vi "Parse GGA Sentence.vi"(7 "date override":timestamp format="%<%x>T", 8 "error in (no error)":errorcluster, 11 "GGA sentence":string) -> (0 "error out":errorcluster, 3 "GGA data":T1 {"DGPS station ID number"."station ID number" min=0.0; "fix quality"."quality" items=["Invalid", "GPS Fix", "DGPS Fix", "PPS Fix", "Real Time Kinematic", "Float RTK", "Estimated", "Manual Input Mode", "Simulation Mode"]; "time of fix"."time (UTC)" format="%^<%.3X\n%x>T"})   [LabVIEW 2017, in "NMEA API.lvlib"]
doc: "Returns data contained in a particular type of NMEA sentence. The input sentence you specify must include valid NMEA formatting and end with a carriage return and line feed, or \\r\\n. You must manually select the polymorphic instance to use."
uses:
  <vilib>/robotics/Protocols/NMEA/NMEA API.lvlib
  <vilib>/robotics/Protocols/NMEA/typedefs/GGA Data.ctl
  <vilib>/robotics/Utilities/NI_Robotics Utilities.lvlib
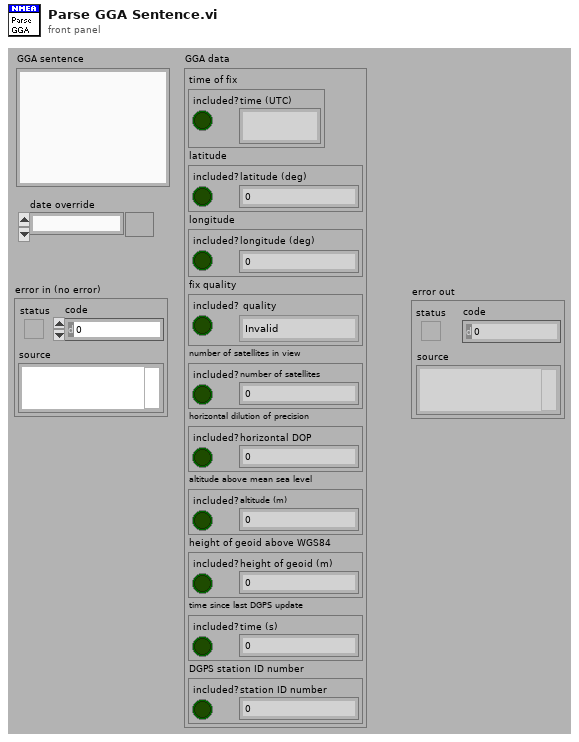
[diagram p1: front panel]
types:
  T1 = typedef "NMEA API.lvlib/GGA Data.ctl" = cluster{"time of fix":cluster{"included?":bool, "time (UTC)":timestamp}, "latitude":cluster{"included?":bool, "latitude (deg)":dbl}, "longitude":cluster{"included?":bool, "longitude (deg)":dbl}, "fix quality":cluster{"included?":bool, "quality":u16}, "number of satellites in view":cluster{"included?":bool, "number of satellites":i8}, "horizontal dilution of precision":cluster{"included?":bool, "horizontal DOP":dbl}, "altitude above mean sea level":cluster{"included?":bool, "altitude (m)":dbl}, "height of geoid above WGS84":cluster{"included?":bool, "height of geoid (m)":dbl}, "time since last DGPS update":cluster{"included?":bool, "time (s)":dbl}, "DGPS station ID number":cluster{"included?":bool, "station ID number":dbl}}
  T2 = cluster{"Valid?":bool, "Number of Satellites":i8}
  T3 = typedef "LVDateTimeRec.ctl" = cluster{"fractional second":dbl, "second":i32, "minute":i32, "hour":i32, "day of month":i32, "month":i32, "year":i32, "day of week":i32, "day of year":i32, "DST":i32}
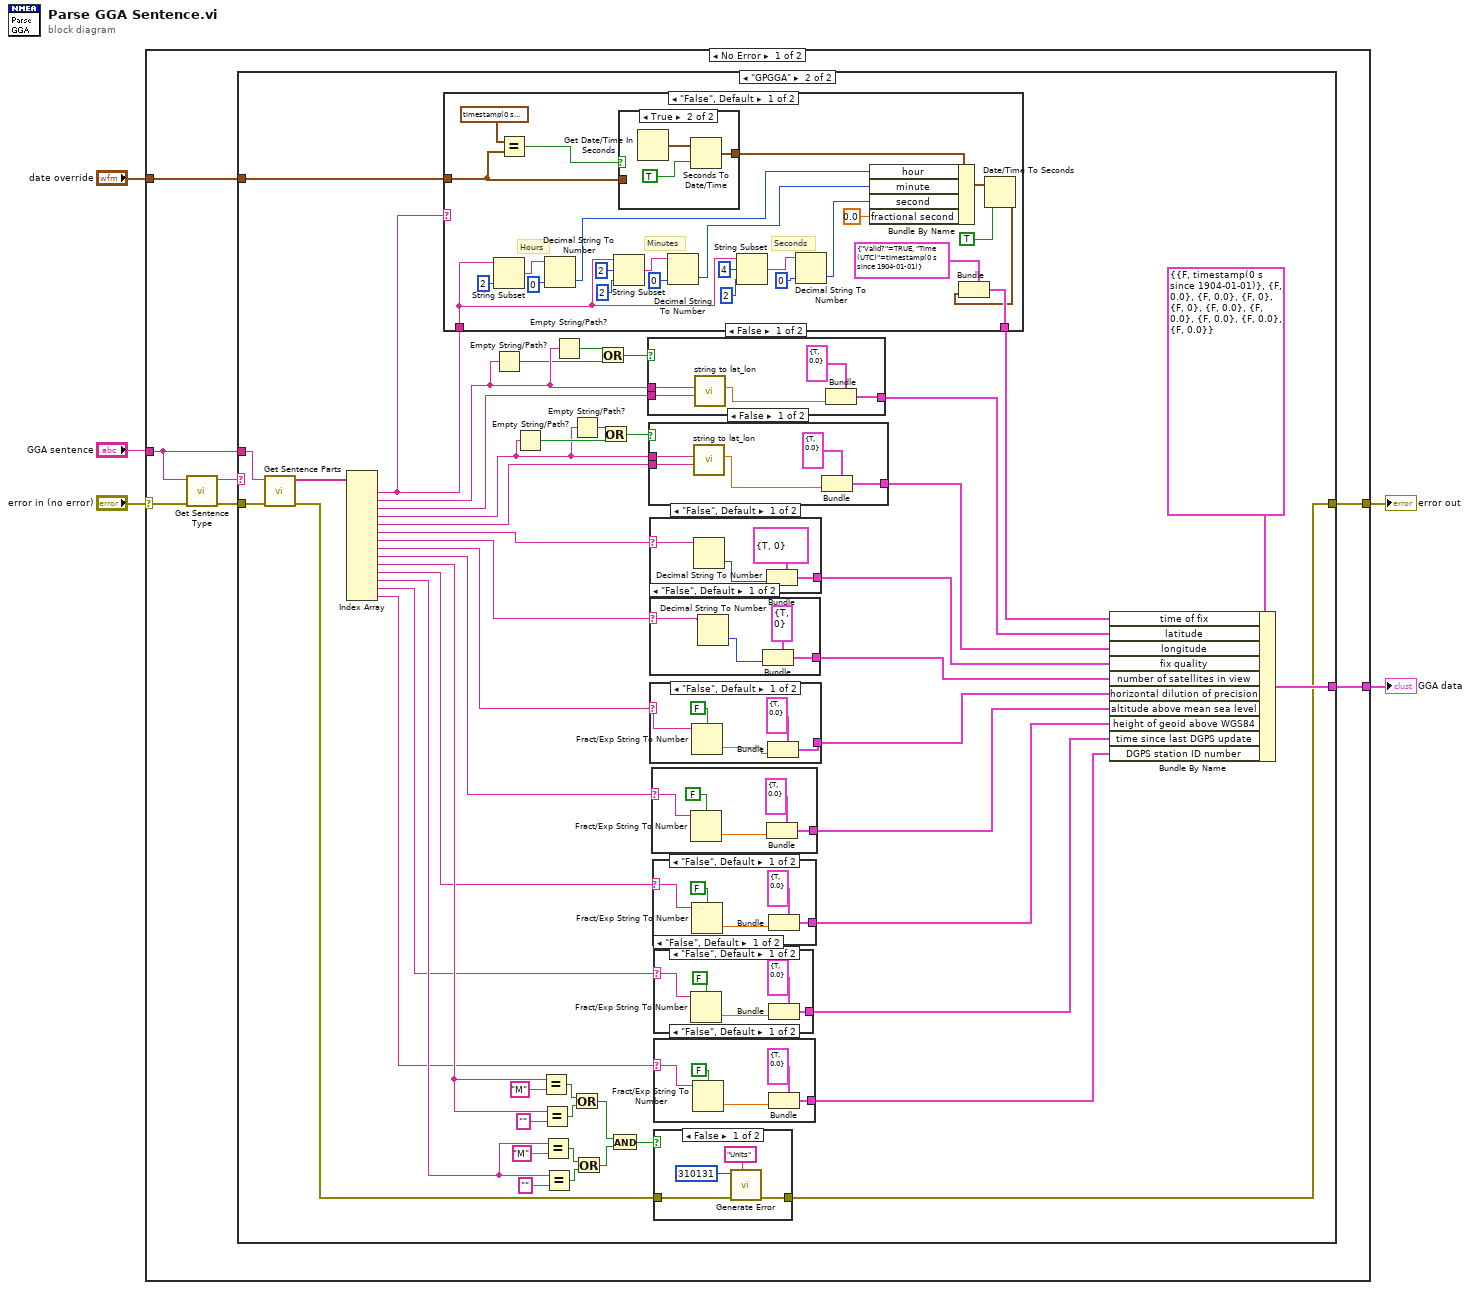
[diagram p0: block diagram]
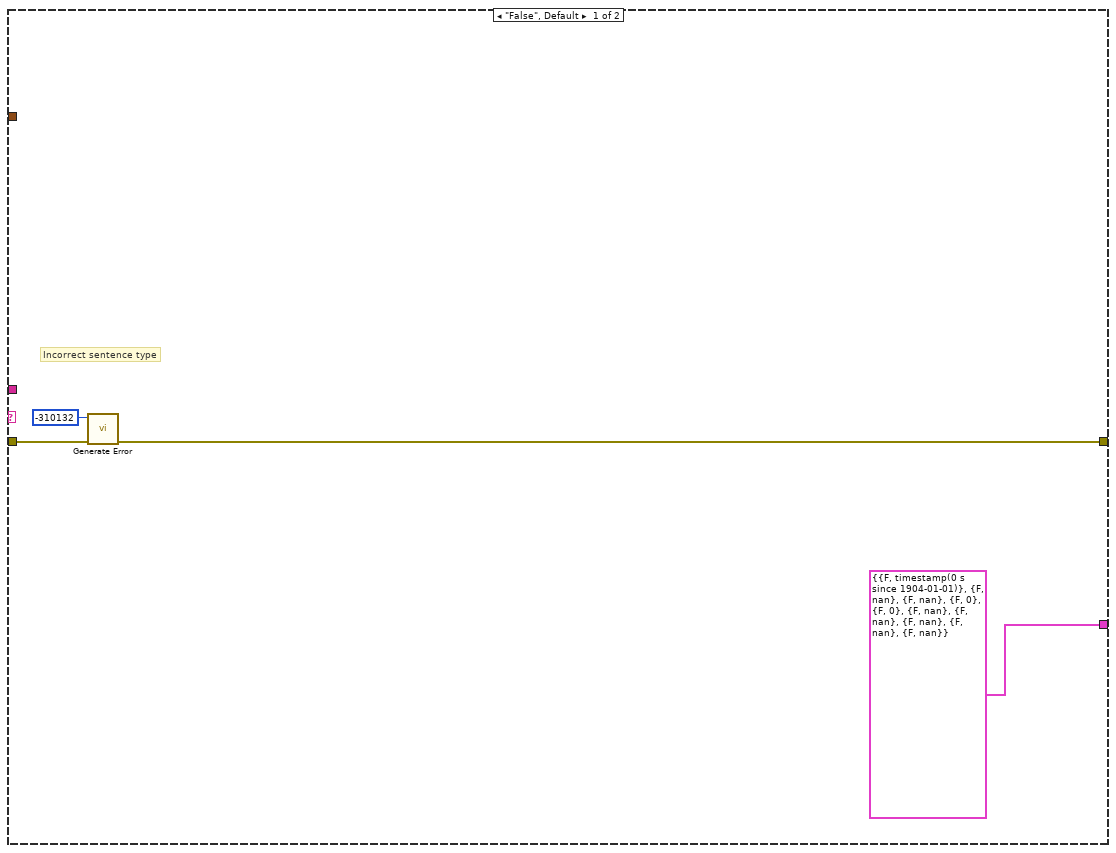
[diagram p2: hidden frame]
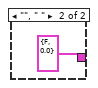
[diagram p4: hidden frame]
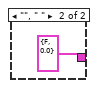
[diagram p5: hidden frame]
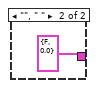
[diagram p6: hidden frame]
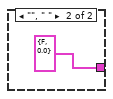
[diagram p7: hidden frame]
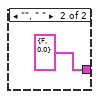
[diagram p8: hidden frame]
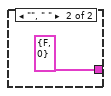
[diagram p9: hidden frame]
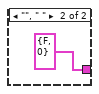
[diagram p10: hidden frame]
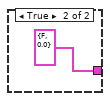
[diagram p11: hidden frame]
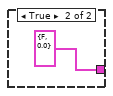
[diagram p12: hidden frame]
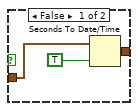
[diagram p13: hidden frame]
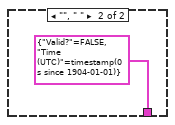
[diagram p14: hidden frame]
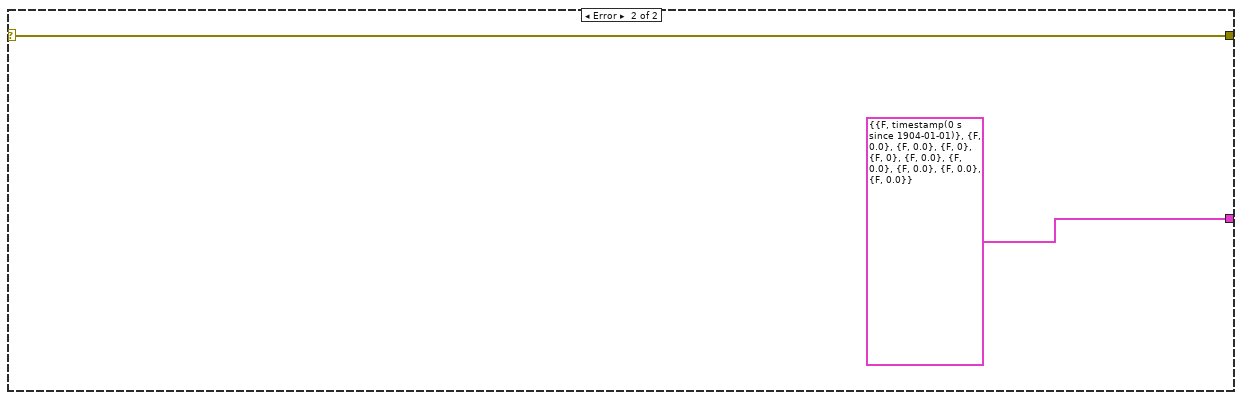
[diagram p15: hidden frame]
diagram:
  n1 = case shown="No Error" "error in (no error)" {
    selector: "error in (no error)" -> [w9 w156]
    tunnel: [w10 w156] -> w3
    tunnel: [w12 T1 {"time of fix"={"included?"=FALSE, "time (UTC)"=timestamp(0 s since 1904-01-01)}, "latitude"={"included?"=FALSE, "latitude (deg)"=0.0}, "longitude"={"included?"=FALSE, "longitude (deg)"=0.0}, "fix quality"={"included?"=FALSE, "quality"=0}, "number of satellites in view"={"included?"=FALSE, "number of satellites"=0}, "horizontal dilution of precision"={"included?"=FALSE, "horizontal DOP"=0.0}, "altitude above mean sea level"={"included?"=FALSE, "altitude (m)"=0.0}, "height of geoid above WGS84"={"included?"=FALSE, "height of geoid (m)"=0.0}, "time since last DGPS update"={"included?"=FALSE, "time (s)"=0.0}, "DGPS station ID number"={"included?"=FALSE, "station ID number"=0.0}} ("GGA Data")] -> w2
    tunnel: "GGA sentence" -> [w7 _]
    tunnel: "date override" -> [w11 _]
    frame No Error {
      n2 = call <vilib>:"Get Sentence Type.vi"("error in (no error)"=w9, "sentence"=w7) -> ("error out"=w8:errorcluster, "sentence type"=w6:string)  [unwired: 1 in, 7 out]
      n3 = case shown="\"GPGGA\"" w6 {
        tunnel: [T1 {"time of fix"={"included?"=FALSE, "time (UTC)"=timestamp(0 s since 1904-01-01)}, "latitude"={"included?"=FALSE, "latitude (deg)"=nan}, "longitude"={"included?"=FALSE, "longitude (deg)"=nan}, "fix quality"={"included?"=FALSE, "quality"=0}, "number of satellites in view"={"included?"=FALSE, "number of satellites"=0}, "horizontal dilution of precision"={"included?"=FALSE, "horizontal DOP"=nan}, "altitude above mean sea level"={"included?"=FALSE, "altitude (m)"=nan}, "height of geoid above WGS84"={"included?"=FALSE, "height of geoid (m)"=nan}, "time since last DGPS update"={"included?"=FALSE, "time (s)"=nan}, "DGPS station ID number"={"included?"=FALSE, "station ID number"=nan}} ("GGA Data") w65] -> w12
        tunnel: w7 -> [_ w18]
        tunnel: w8 -> [w14 w64]
        tunnel: w11 -> [_ w63]
        tunnel: [w13 w42] -> w10
        frame "False", Default {
          # "Incorrect sentence type"
          n4 = call <vilib>:"Generate Error.vi"("error in (no error)"=w14, "code"=-310132) -> ("error out"=w13:errorcluster)  [unwired: 9 in]
        }
        frame "GPGGA" {
          n5 = call <vilib>:"Get Sentence Parts.vi"("error in (no error)"=w64, "sentence"=w18) -> ("error out"=w46:errorcluster, "sentence data"=w17:string[])  [unwired: 1 in, 7 out]
          n6 = Index Array(array=w17) -> (element #1=w26:string, element #2=w58:string, element #3=w62:string, element #4=w54:string, element #5=w61:string, element #6=w25:string, element #7=w24:string, element #8=w23:string, element #9=w22:string, element #10=w41:string, element #11=w21:string, element #12=w35:string, element #13=w20:string, element #14=w19:string)  [unwired: 14 in]
          n7 = case shown="\"False\", Default" w26 {
            tunnel: w63 -> [w145 _]
            tunnel: [w129 cluster{"Valid?":bool, "Time (UTC)":timestamp} {"Valid?"=FALSE, "Time (UTC)"=timestamp(0 s since 1904-01-01)} ("Time of Fix")] -> w52
            tunnel: w26 -> [w130 _]
            frame "False", Default {
              # "Seconds"
              # "Minutes"
              # "Hours"
              n8 = String Subset(string=w130, length (rest)=2 ("length (rest)")) -> (substring=w137:string)  [unwired: 1 out]
              n9 = Equal?(x=timestamp(0 s since 1904-01-01), y=w145) -> (x = y?=w147:bool)
              n10 = Decimal String To Number(string=w137, default (0L)=0 ("default (0 DBL)")) -> (number=w131:i32)  [unwired: 2 out]
              n11 = String Subset(string=w130, offset (0)=2, length (rest)=2 ("length (rest)")) -> (substring=w138:string)
              n12 = case shown="True" w147 {
                tunnel: w145 -> [w150 _]
                tunnel: [w149 w152] -> w135
                frame False {
                  n13 = Seconds To Date/Time(time stamp (now)=w150, to UTC (F)=TRUE) -> (date time rec=w149:T3)
                }
                frame True {
                  n14 = Get Date/Time In Seconds() -> (seconds since 1Jan1904=w153:timestamp)
                  n15 = Seconds To Date/Time(time stamp (now)=w153, to UTC (F)=TRUE) -> (date time rec=w152:T3)
                }
              }
              n16 = Decimal String To Number(string=w138, default (0L)=0 ("default (0 DBL)")) -> (number=w132:i32)  [unwired: 2 out]
              n17 = String Subset(string=w130, offset (0)=4, length (rest)=2 ("length (rest)")) -> (substring=w141:string)
              n18 = Decimal String To Number(string=w141, default (0L)=0 ("default (0 DBL)")) -> (number=w133:i32)  [unwired: 2 out]
              n19 = Bundle By Name(cluster=w135, "hour"=w131, "minute"=w132, "second"=w133, "fractional second"=0.0) -> (w134:T3)
              n20 = Date/Time To Seconds(1:TRUE, 2:w134) -> (0:w127:timestamp)
              n21 = Bundle(cluster=cluster{"Valid?":bool, "Time (UTC)":timestamp} {"Valid?"=TRUE, "Time (UTC)"=timestamp(0 s since 1904-01-01)} ("Time of Fix"), "Time (UTC)"=w127) -> (w129:cluster{"Valid?":bool, "Time (UTC)":timestamp})  [unwired: 1 out]
            }
            frame "", " " {
            }
          }
          n22 = Empty String/Path?(string/path=w58) -> (empty?=w57:bool)
          n23 = Empty String/Path?(string/path=w54) -> (empty?=w56:bool)
          n24 = Equal?(x=w41, y="M") -> (x = y?=w44:bool)
          n25 = Equal?(x=w41, y="") -> (x = y?=w45:bool)
          n26 = Equal?(x=w35, y="M") -> (x = y?=w37:bool)
          n27 = Equal?(x=w35, y="") -> (x = y?=w36:bool)
          n28 = Empty String/Path?(string/path=w58) -> (empty?=w59:bool)
          n29 = Empty String/Path?(string/path=w54) -> (empty?=w55:bool)
          n30 = Or(x=w44, y=w45) -> (x .or. y?=w33:bool)
          n31 = Or(x=w37, y=w36) -> (x .or. y?=w32:bool)
          n32 = Or(x=w59, y=w57) -> (x .or. y?=w60:bool)
          n33 = Or(x=w55, y=w56) -> (x .or. y?=w53:bool)
          n34 = And(x=w33, y=w32) -> (x .and. y?=w34:bool)
          n35 = case shown="False" w60 {
            tunnel: [w119 cluster{"Valid?":bool, "Latitude (Deg)":dbl} {"Valid?"=FALSE, "Latitude (Deg)"=0.0} ("Latitude")] -> w49
            tunnel: w58 -> [w121 _]
            tunnel: w62 -> [w120 _]
            frame False {
              n36 = call <vilib>:"string to lat_lon.vi"("direction string"=w120, "numeric string for lat/lon"=w121) -> ("composite value"=w117:dbl)  [unwired: 1 in, 8 out]
              n37 = Bundle(cluster=cluster{"Valid?":bool, "Latitude (Deg)":dbl} {"Valid?"=TRUE, "Latitude (Deg)"=0.0} ("Latitude"), "Latitude (Deg)"=w117) -> (w119:cluster{"Valid?":bool, "Latitude (Deg)":dbl})  [unwired: 1 out]
            }
            frame True {
            }
          }
          n38 = case shown="False" w53 {
            tunnel: w61 -> [w115 _]
            tunnel: w54 -> [w114 _]
            tunnel: [w111 cluster{"Valid?":bool, "Longitude (Deg)":dbl} {"Valid?"=FALSE, "Longitude (Deg)"=0.0} ("Longitude")] -> w47
            frame False {
              n39 = call <vilib>:"string to lat_lon.vi"("direction string"=w115, "numeric string for lat/lon"=w114) -> ("composite value"=w113:dbl)  [unwired: 1 in, 8 out]
              n40 = Bundle(cluster=cluster{"Valid?":bool, "Longitude (Deg)":dbl} {"Valid?"=TRUE, "Longitude (Deg)"=0.0} ("Longitude"), "Longitude (Deg)"=w113) -> (w111:cluster{"Valid?":bool, "Longitude (Deg)":dbl})  [unwired: 1 out]
            }
            frame True {
            }
          }
          n41 = case shown="\"False\", Default" w25 {
            selector: w25 -> [w106 _]
            tunnel: [w107 cluster{"Valid?":bool, "Fix Quality":u16} {"Valid?"=FALSE, "Fix Quality"=0} ("Fix Quality")] -> w51
            frame "False", Default {
              n42 = Decimal String To Number(string=w106) -> (number=w108:i32)  [unwired: 3 out]
              n43 = Bundle(cluster=cluster{"Valid?":bool, "Fix Quality":u16} {"Valid?"=TRUE, "Fix Quality"=0} ("Fix Quality"), "Fix Quality"=w108) -> (w107:cluster{"Valid?":bool, "Fix Quality":u16})  [unwired: 1 out]
            }
            frame "", " " {
            }
          }
          n44 = case shown="\"False\", Default" w24 {
            selector: w24 -> [w101 _]
            tunnel: [w102 T2 {"Valid?"=FALSE, "Number of Satellites"=0} ("Number of Satellites Being Tracked")] -> w50
            frame "False", Default {
              n45 = Decimal String To Number(string=w101) -> (number=w104:i32)  [unwired: 3 out]
              n46 = Bundle(cluster=T2 {"Valid?"=TRUE, "Number of Satellites"=0} ("Number of Satellites Being Tracked"), "Number of Satellites"=w104) -> (w102:T2)  [unwired: 1 out]
            }
            frame "", " " {
            }
          }
          n47 = case shown="\"False\", Default" w23 {
            selector: w23 -> [w96 _]
            tunnel: [w97 cluster{"Valid?":bool, "Horizontal DOP":dbl} {"Valid?"=FALSE, "Horizontal DOP"=0.0} ("Horizontal Dilution of Precision")] -> w31
            frame "False", Default {
              n48 = Fract/Exp String To Number(use system decimal point (T)=FALSE, string=w96) -> (number=w98:dbl)  [unwired: 3 out]
              n49 = Bundle(cluster=cluster{"Valid?":bool, "Horizontal DOP":dbl} {"Valid?"=TRUE, "Horizontal DOP"=0.0} ("Horizontal Dilution of Precision"), "Horizontal DOP"=w98) -> (w97:cluster{"Valid?":bool, "Horizontal DOP":dbl})  [unwired: 1 out]
            }
            frame "", " " {
            }
          }
          n50 = case shown="\"False\", Default" w22 {
            selector: w22 -> [w90 _]
            tunnel: [w91 cluster{"Valid?":bool, "Horizontal DOP":dbl} {"Valid?"=FALSE, "Horizontal DOP"=0.0} ("Horizontal Dilution of Precision")] -> w30
            frame "False", Default {
              n51 = Fract/Exp String To Number(use system decimal point (T)=FALSE, string=w90) -> (number=w92:dbl)  [unwired: 3 out]
              n52 = Bundle(cluster=cluster{"Valid?":bool, "Horizontal DOP":dbl} {"Valid?"=TRUE, "Horizontal DOP"=0.0} ("Horizontal Dilution of Precision"), "Horizontal DOP"=w92) -> (w91:cluster{"Valid?":bool, "Horizontal DOP":dbl})  [unwired: 1 out]
            }
            frame "", " " {
            }
          }
          n53 = case shown="\"False\", Default" w21 {
            selector: w21 -> [w84 _]
            tunnel: [w85 cluster{"Valid?":bool, "Horizontal DOP":dbl} {"Valid?"=FALSE, "Horizontal DOP"=0.0} ("Horizontal Dilution of Precision")] -> w29
            frame "False", Default {
              n54 = Fract/Exp String To Number(use system decimal point (T)=FALSE, string=w84) -> (number=w86:dbl)  [unwired: 3 out]
              n55 = Bundle(cluster=cluster{"Valid?":bool, "Horizontal DOP":dbl} {"Valid?"=TRUE, "Horizontal DOP"=0.0} ("Horizontal Dilution of Precision"), "Horizontal DOP"=w86) -> (w85:cluster{"Valid?":bool, "Horizontal DOP":dbl})  [unwired: 1 out]
            }
            frame "", " " {
            }
          }
          n56 = case shown="\"False\", Default" w20 {
            selector: w20 -> [w78 _]
            tunnel: [w79 cluster{"Valid?":bool, "Horizontal DOP":dbl} {"Valid?"=FALSE, "Horizontal DOP"=0.0} ("Horizontal Dilution of Precision")] -> w28
            frame "False", Default {
              n57 = Fract/Exp String To Number(use system decimal point (T)=FALSE, string=w78) -> (number=w80:dbl)  [unwired: 3 out]
              n58 = Bundle(cluster=cluster{"Valid?":bool, "Horizontal DOP":dbl} {"Valid?"=TRUE, "Horizontal DOP"=0.0} ("Horizontal Dilution of Precision"), "Horizontal DOP"=w80) -> (w79:cluster{"Valid?":bool, "Horizontal DOP":dbl})  [unwired: 1 out]
            }
            frame "", " " {
            }
          }
          n59 = case shown="\"False\", Default" w19 {
            selector: w19 -> [w72 _]
            tunnel: [w73 cluster{"Valid?":bool, "Horizontal DOP":dbl} {"Valid?"=FALSE, "Horizontal DOP"=0.0} ("Horizontal Dilution of Precision")] -> w27
            frame "False", Default {
              n60 = Fract/Exp String To Number(use system decimal point (T)=FALSE, string=w72) -> (number=w74:dbl)  [unwired: 3 out]
              n61 = Bundle(cluster=cluster{"Valid?":bool, "Horizontal DOP":dbl} {"Valid?"=TRUE, "Horizontal DOP"=0.0} ("Horizontal Dilution of Precision"), "Horizontal DOP"=w74) -> (w73:cluster{"Valid?":bool, "Horizontal DOP":dbl})  [unwired: 1 out]
            }
            frame "", " " {
            }
          }
          n62 = case shown="False" w34 {
            tunnel: w46 -> [w68 w70]
            tunnel: [w67 w70] -> w42
            frame False {
              n63 = call <vilib>:"Generate Error.vi"("<append> (\"\")"="Units" ("<append> (\"\")"), "error in (no error)"=w68, "code"=310131) -> ("error out"=w67:errorcluster)  [unwired: 8 in]
            }
            frame True {
            }
          }
          n64 = Bundle By Name(cluster=T1 {"time of fix"={"included?"=FALSE, "time (UTC)"=timestamp(0 s since 1904-01-01)}, "latitude"={"included?"=FALSE, "latitude (deg)"=0.0}, "longitude"={"included?"=FALSE, "longitude (deg)"=0.0}, "fix quality"={"included?"=FALSE, "quality"=0}, "number of satellites in view"={"included?"=FALSE, "number of satellites"=0}, "horizontal dilution of precision"={"included?"=FALSE, "horizontal DOP"=0.0}, "altitude above mean sea level"={"included?"=FALSE, "altitude (m)"=0.0}, "height of geoid above WGS84"={"included?"=FALSE, "height of geoid (m)"=0.0}, "time since last DGPS update"={"included?"=FALSE, "time (s)"=0.0}, "DGPS station ID number"={"included?"=FALSE, "station ID number"=0.0}} ("GGA Data"), "time of fix"=w52, "latitude"=w49, "longitude"=w47, "fix quality"=w51, "number of satellites in view"=w50, "horizontal dilution of precision"=w31, "altitude above mean sea level"=w30, "height of geoid above WGS84"=w29, "time since last DGPS update"=w28, "DGPS station ID number"=w27) -> (w65:T1)
        }
      }
    }
    frame Error {
    }
  }
  "error out" <- w3
  "GGA data" <- w2
